vi "Main.vi"() -> ()   [LabVIEW 2020]
doc: "Machine d'état simple"
uses:
  Control/Ctrl_states.ctl
  Control/Ctrl_local.ctl
panel:
  in  "Btn_Stop":bool
  in  "Btn_Error":bool
  out "error out":errorcluster caption="sortie d'erreur"
  in  "error in":errorcluster caption="entrée d'erreur"
  out "Display_char":string
  out "Display_Bool":bool
  in  "Btn_Etat3":bool
  in  "Btn_Etat2":bool
  in  "Btn_Etat1":bool
  # "State machine"
  # "Commandes"
  # "Indicateurs"
  # "Error command"
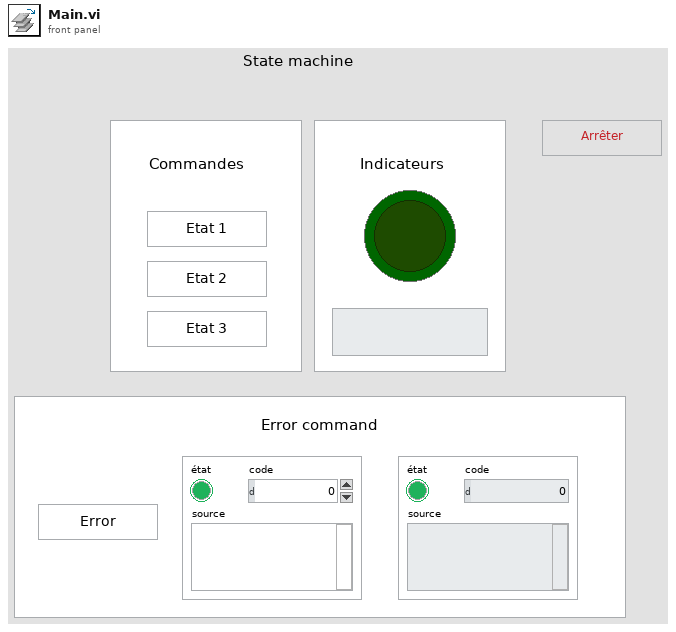
[diagram p1: front panel]
types:
  T1 = typedef "Ctrl_states.ctl" = enum16{"Initialisation", "Idle", "Stop", "Error", "Display", "Etat 1", "Etat 2", "Etat 3"}
  T2 = typedef "Ctrl_local.ctl" = cluster{"Bool":bool, "Char":string}
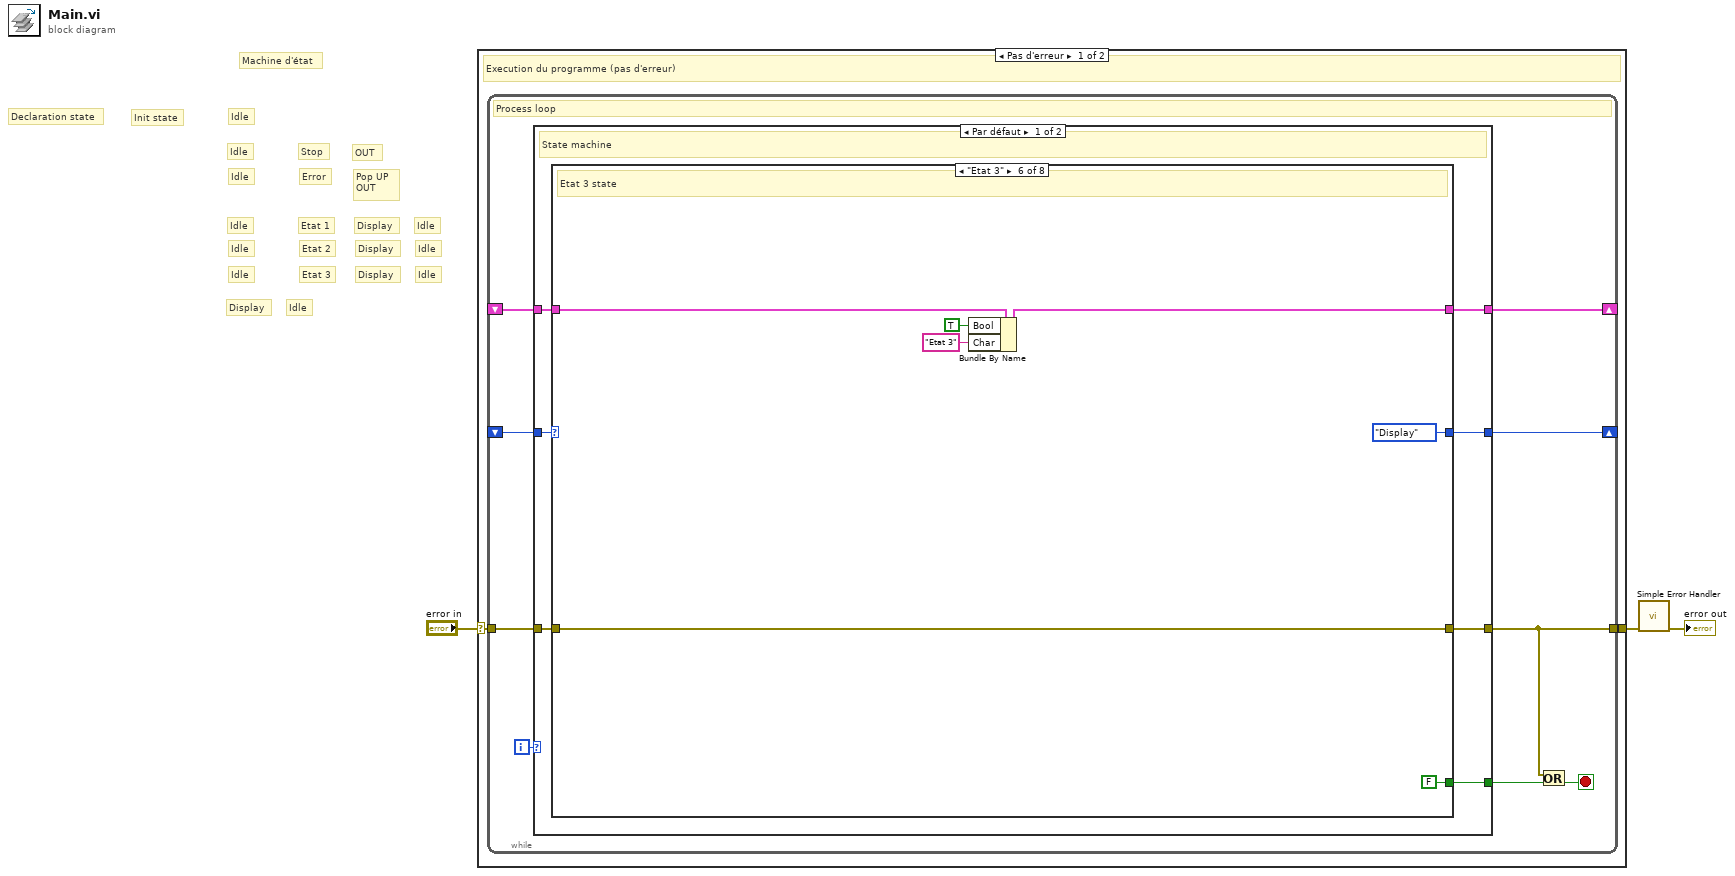
[diagram p0: block diagram]
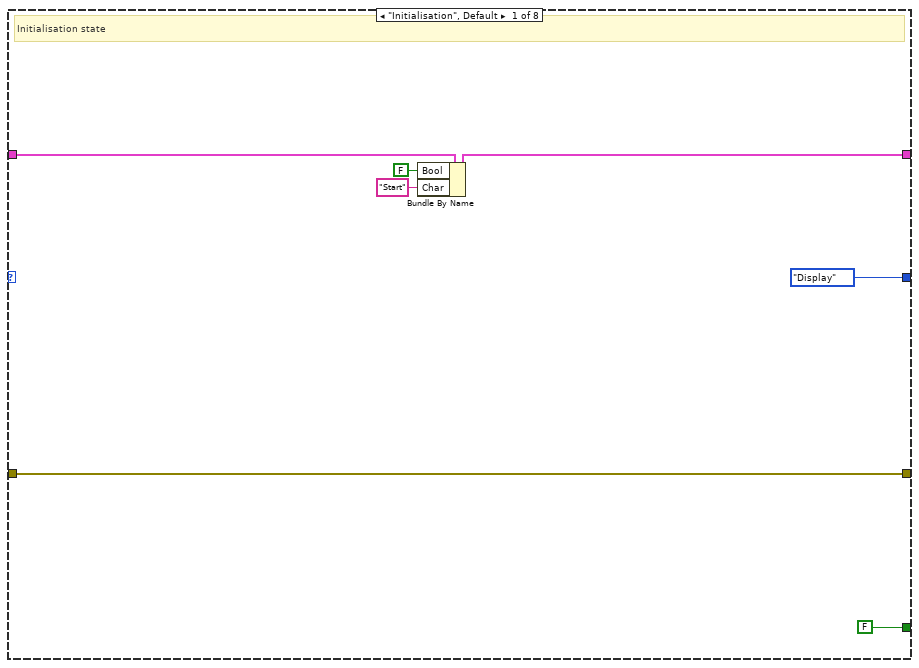
[diagram p2: hidden frame]
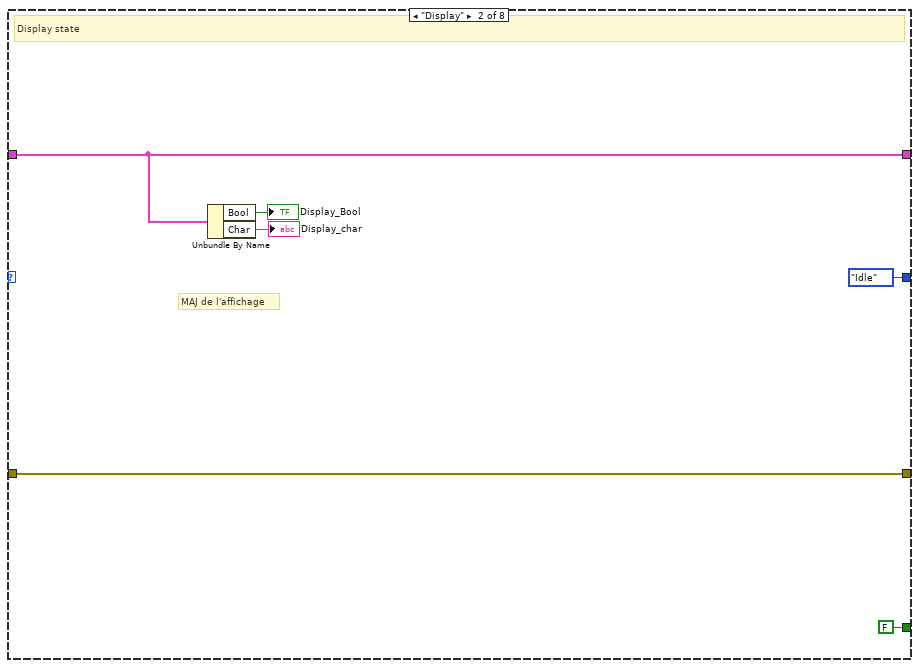
[diagram p3: hidden frame]
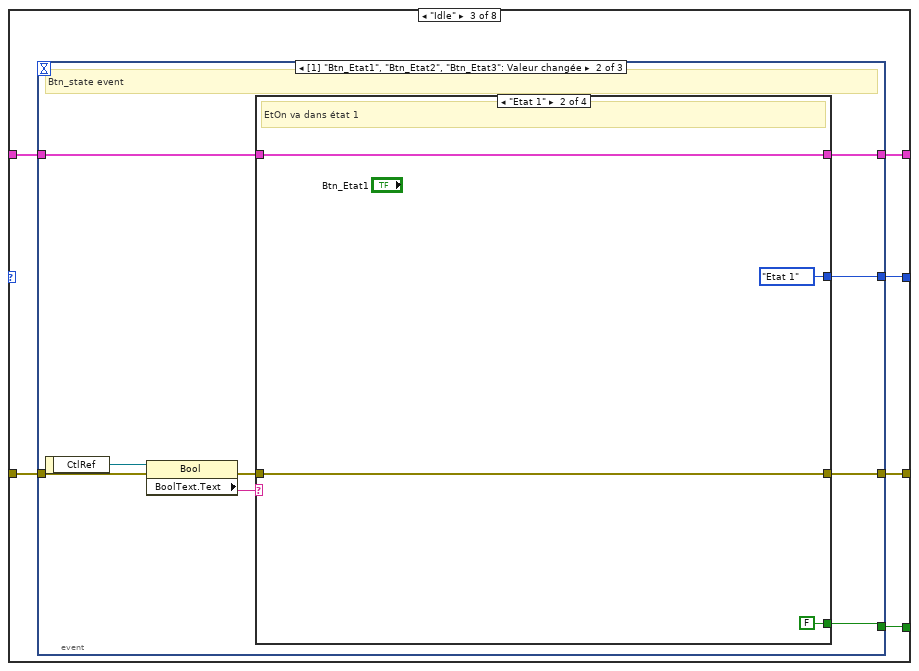
[diagram p4: hidden frame]
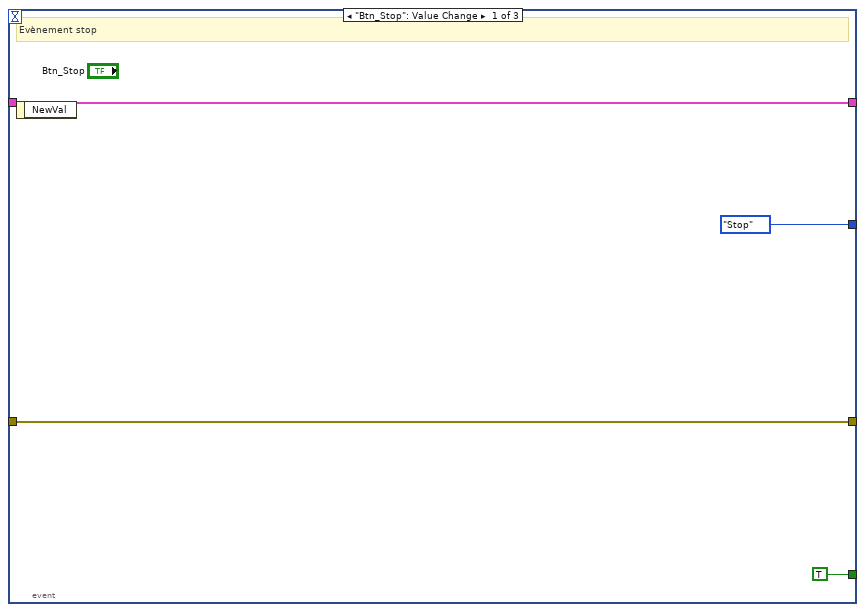
[diagram p5: hidden frame]
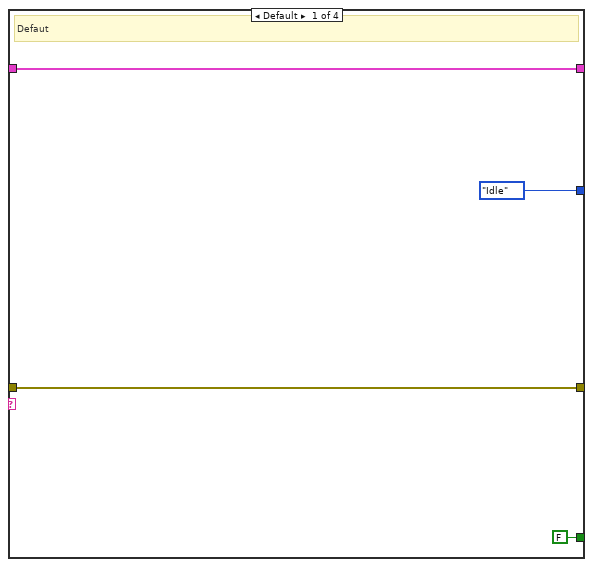
[diagram p6: hidden frame]
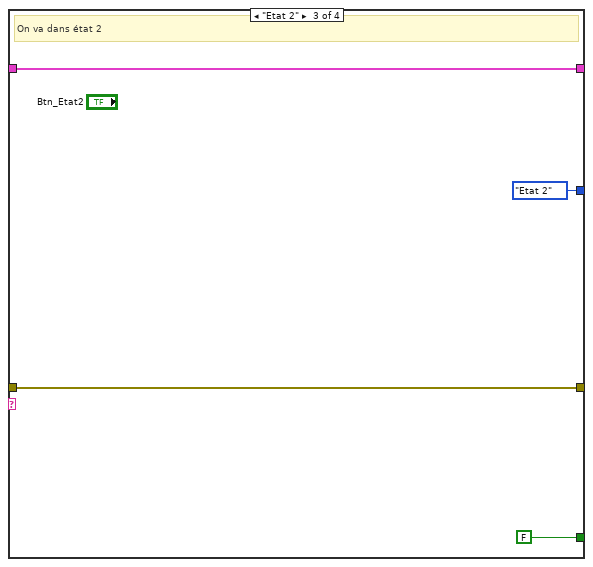
[diagram p7: hidden frame]
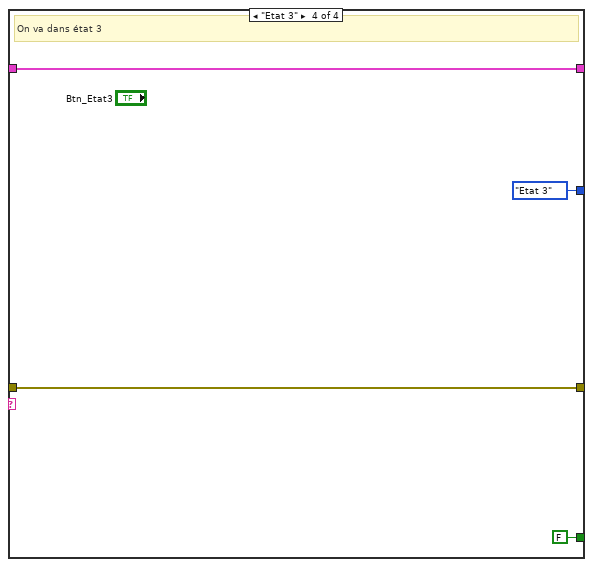
[diagram p8: hidden frame]
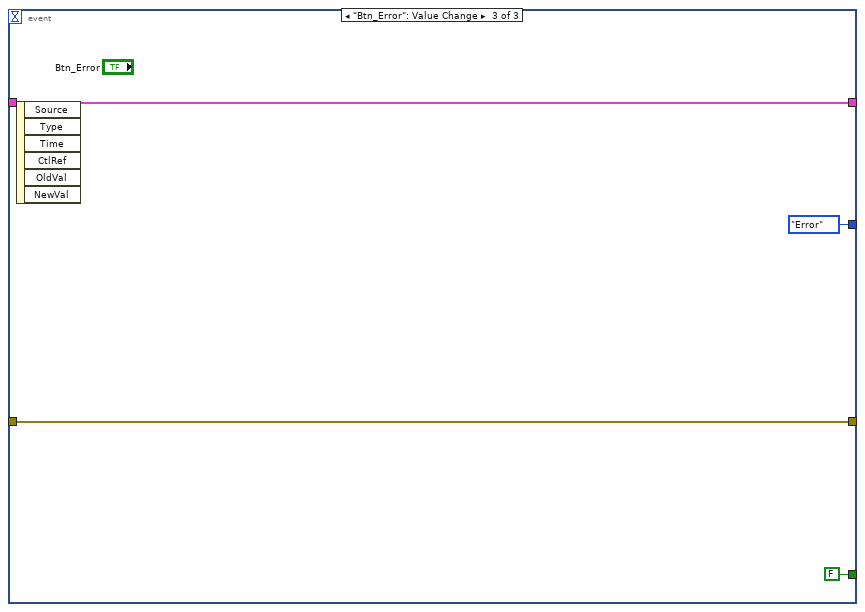
[diagram p9: hidden frame]
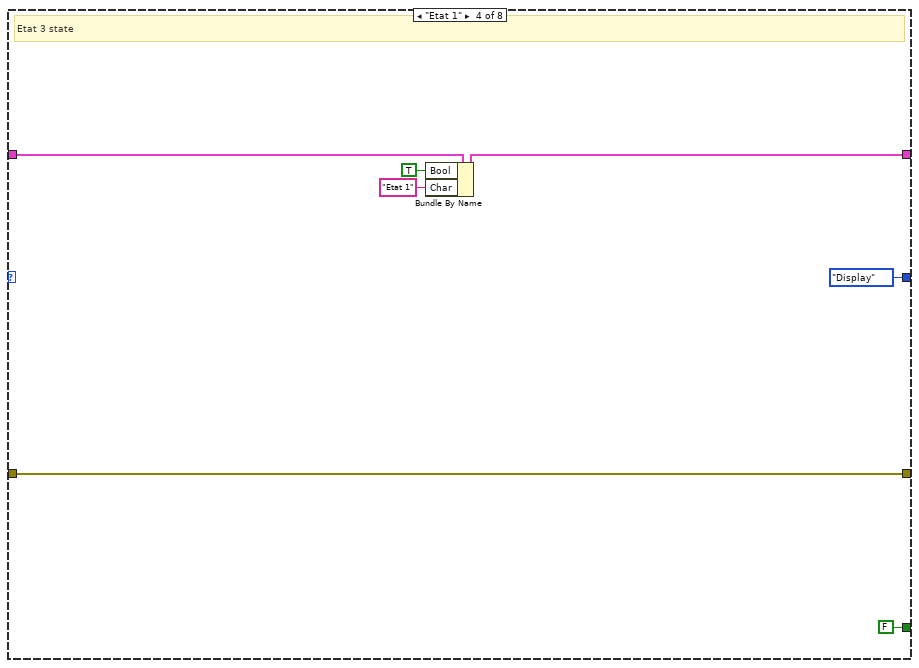
[diagram p10: hidden frame]
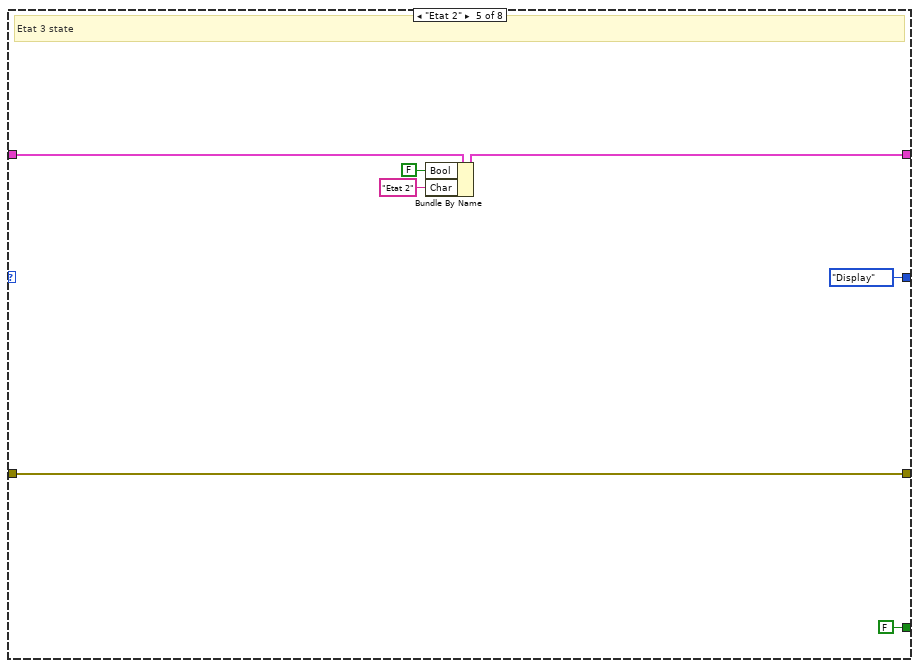
[diagram p11: hidden frame]
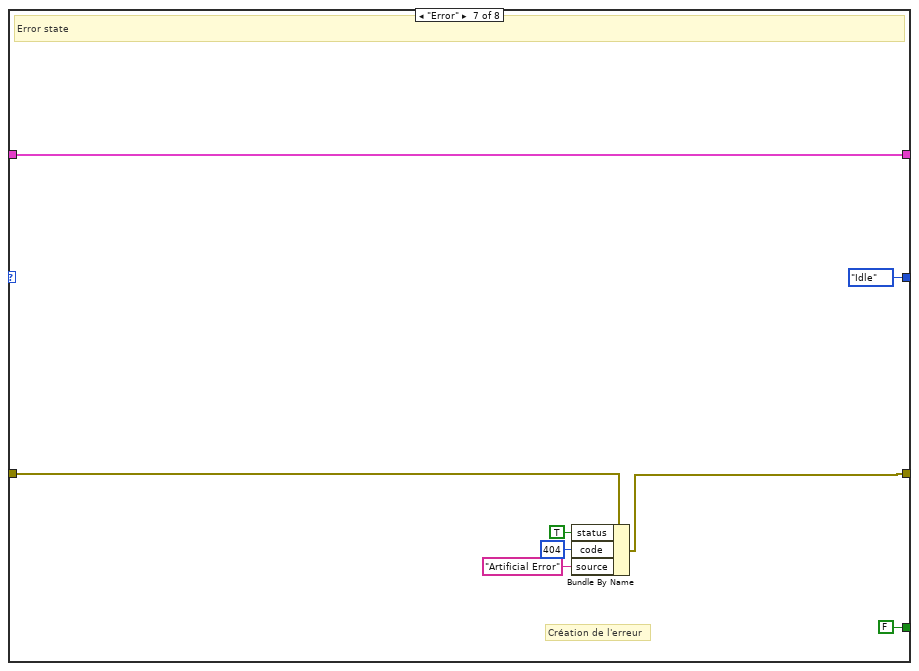
[diagram p12: hidden frame]
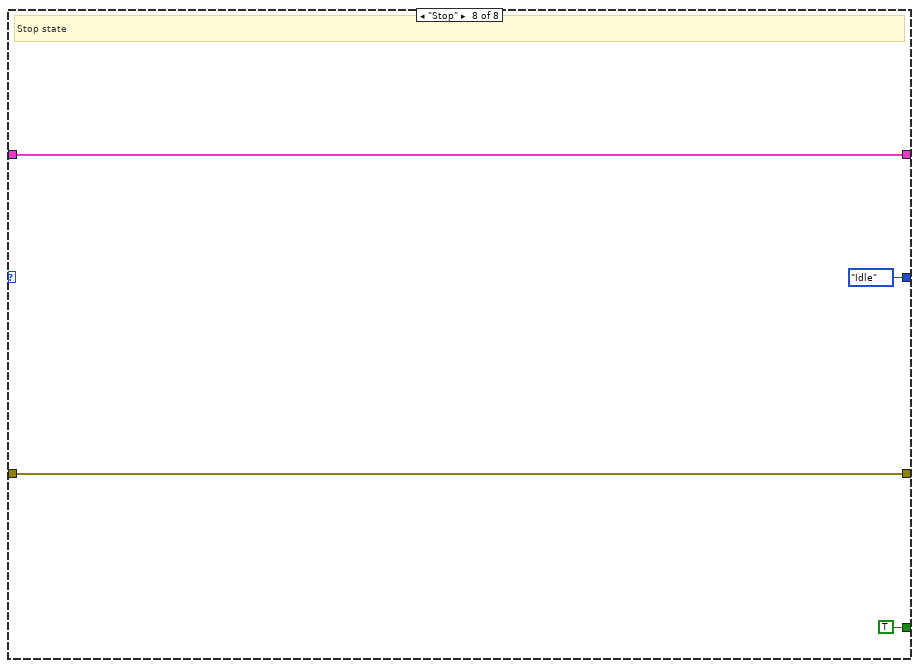
[diagram p13: hidden frame]
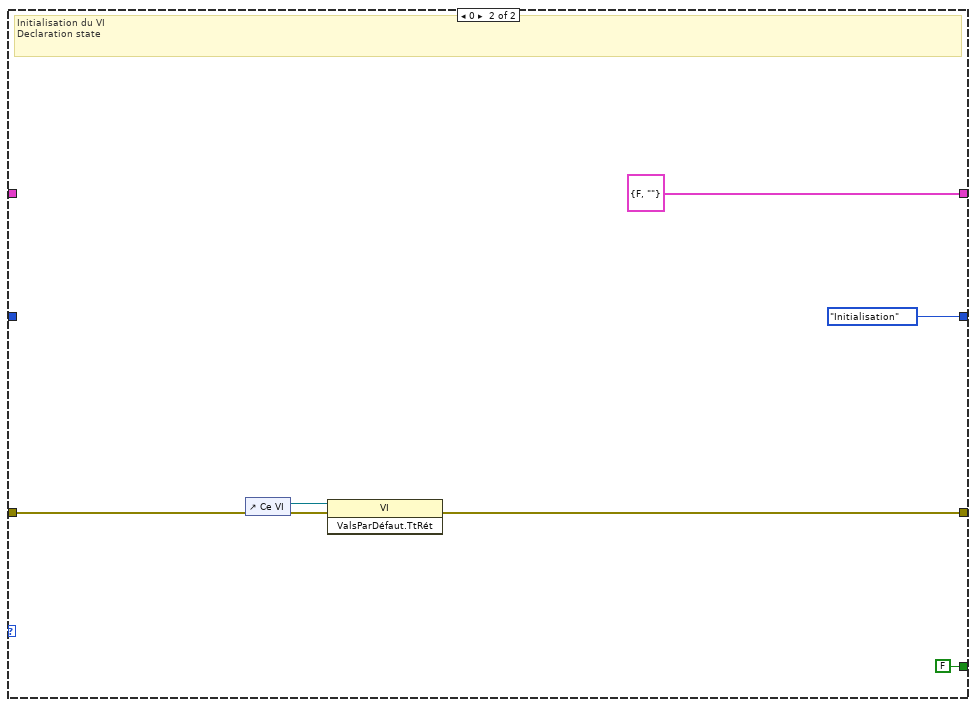
[diagram p14: hidden frame]
diagram:
  # "Idle"
  # "Display"
  # "Idle"
  # "Display"
  # "Etat 3"
  # "Idle"
  # "Idle"
  # "Display"
  # "Etat 2"
  # "Idle"
  # "Idle"
  # "Display"
  # "Etat 1"
  # "Idle"
  # "Pop UP \nOUT"
  # "Error"
  # "Idle"
  # "OUT"
  # "Stop"
  # "Idle"
  # "Idle"
  # "Init state"
  # "Declaration state"
  # "Machine d'état"
  n1 = case shown="Pas d'erreur" "error in" {
    selector: "error in" -> [w5 w113]
    tunnel: [w4 w113] -> w2
    frame No Error {
      # "Execution du programme (pas d'erreur)"
      n2 = while {
        tunnel: w5 -> [w14]
        tunnel: [w8] -> w4
        shift-right: [w12] -> _
        shift-left: _ -> [w11]
        shift-right: [w7] -> _
        shift-left: _ -> [w6]
        i -> [w13]
        stop <- w9 stop-if-true
        # "Process loop"
        n3 = case shown="Par défaut" w13 {
          tunnel: w14 -> [w19 w111]
          tunnel: [w17 w110] -> w8
          tunnel: [w20 Ctrl_states."Initialisation" ("State")] -> w12
          tunnel: w11 -> [w21 _]
          tunnel: [w18 FALSE] -> w10
          tunnel: [w15 T2 {"Bool"=FALSE, "Char"=""} ("Local")] -> w7
          tunnel: w6 -> [w16 _]
          frame Default {
            # "State machine"
            n4 = case shown="\"Etat 3\"" w21 {
              tunnel: [Ctrl_states."Display" ("State") Ctrl_states."Idle" ("State") w35 Ctrl_states."Display" ("State") Ctrl_states."Display" ("State") Ctrl_states."Display" ("State") Ctrl_states."Idle" ("State") Ctrl_states."Idle" ("State")] -> w20
              tunnel: w19 -> [w26 w31 w40 w78 w85 w92 w100 w106]
              tunnel: [FALSE FALSE w39 FALSE FALSE FALSE FALSE TRUE] -> w18
              tunnel: [w26 w31 w38 w78 w85 w92 w99 w106] -> w17
              tunnel: w16 -> [w25 w34 w37 w80 w87 w94 w95 w103]
              tunnel: [w24 w34 w36 w76 w83 w90 w95 w103] -> w15
              frame "Initialisation", Default {
                # "Initialisation state"
                n5 = Bundle By Name(cluster=w25, "Bool"=FALSE, "Char"="Start") -> (w24:T2)
              }
              frame "Display" {
                # "MAJ de l'affichage"
                # "Display state"
                n6 = Unbundle By Name(w34) -> ("Bool"=→"Display_Bool":bool, "Char"=→"Display_char":string)
              }
              frame "Idle" {
                n7 = event shown="[1] \"Btn_Etat1\", \"Btn_Etat2\", \"Btn_Etat3\": Valeur changée" {
                  selector: _ -> [_ _ _]
                  dyn-events: _ -> [_ _ _]
                  timeout: _ -> [_ _ _]
                  tunnel: w40 -> [w43 w52 w73]
                  tunnel: [TRUE w45 FALSE] -> w39
                  tunnel: [w43 w46 w73] -> w38
                  tunnel: w37 -> [w42 w50 w71]
                  tunnel: [w42 w49 w71] -> w36
                  tunnel: [Ctrl_states."Stop" ("State") w48 Ctrl_states."Error" ("State")] -> w35
                  event "Btn_Stop": Value Change {
                    # "Evènement stop"
                    n8 = event-data() -> ()  [unwired: 1 in, 1 out]
                  }
                  event "Btn_Etat1", "Btn_Etat2", "Btn_Etat3": Value Change {
                    # "Btn_state event"
                    n9 = event-data() -> ("CtlRef"=w53:refnum<vi>)  [unwired: 1 in]
                    n10 = property class="Bool"(reference=w53, error in=w52) -> (error out=w47:errorcluster, "BoolText.Text"=w51:string)  [unwired: 1 out]
                    n11 = case shown="\"Etat 1\"" w51 {
                      tunnel: w50 -> [w57 w61 w65 w69]
                      tunnel: [w57 w61 w65 w69] -> w49
                      tunnel: [Ctrl_states."Idle" ("State") Ctrl_states."Etat 1" ("State") Ctrl_states."Etat 2" ("State") Ctrl_states."Etat 3" ("State")] -> w48
                      tunnel: w47 -> [w55 w59 w63 w67]
                      tunnel: [w55 w59 w63 w67] -> w46
                      tunnel: [FALSE FALSE FALSE FALSE] -> w45
                      frame Default {
                        # "Defaut"
                      }
                      frame "Etat 1" {
                        # "EtOn va dans état 1"
                      }
                      frame "Etat 2" {
                        # "On va dans état 2"
                      }
                      frame "Etat 3" {
                        # "On va dans état 3"
                      }
                    }
                  }
                  event "Btn_Error": Value Change {
                    n12 = event-data() -> ()  [unwired: 1 in, 6 out]
                  }
                }
              }
              frame "Etat 1" {
                # "Etat 3 state"
                n13 = Bundle By Name(cluster=w80, "Bool"=TRUE, "Char"="Etat 1") -> (w76:T2)
              }
              frame "Etat 2" {
                # "Etat 3 state"
                n14 = Bundle By Name(cluster=w87, "Bool"=FALSE, "Char"="Etat 2") -> (w83:T2)
              }
              frame "Etat 3" {
                # "Etat 3 state"
                n15 = Bundle By Name(cluster=w94, "Bool"=TRUE, "Char"="Etat 3") -> (w90:T2)
              }
              frame "Error" {
                # "Création de l'erreur"
                # "Error state"
                n16 = Bundle By Name(cluster=w100, "status"=TRUE, "code"=404, "source"="Artificial Error") -> (w99:errorcluster)
              }
              frame "Stop" {
                # "Stop state"
              }
            }
          }
          frame 0 {
            # "Initialisation du VI\nDeclaration state"
            n17 = control-ref of="Ce VI"() -> (w112:refnum<vi>)
            n18 = invoke class="VI" method="ValsParDéfaut.TtRét"(reference=w112, error in=w111) -> (error out=w110:errorcluster)  [unwired: 1 in, 2 out]
          }
        }
        n19 = Or(x=w8, y=w10) -> (x .or. y?=w9:bool)
      }
    }
    frame Error {
      # "non execution du programme (erreur)"
    }
  }
  n20 = call <vilib>:"Simple Error Handler.vi"("error in (no error)"=w2) -> ("error out"=→"error out":errorcluster)  [unwired: 4 in, 4 out]
